vi "Start Measurement.vi"(8 "error in (no error)":errorcluster, 11 "User Interface in":refnum<class "User Interface.lvclass">) -> (0 "error out":errorcluster, 3 "User Interface out":refnum<class "User Interface.lvclass">)   [LabVIEW 2016, in "User Interface.lvlib" / "User Interface.lvclass"]
uses:
  User Interface.lvclass
  <vilib>/ActorFramework/Actor/Actor.lvclass
  Controllers/Acquisition Controller/Acquisition Controller.lvclass
  Z:/VM Shared Folder/Trace Grabber/Controllers/Abstract Controller/Abstract Controller.lvclass
  C:/Program Files (x86)/National Instruments/LabVIEW 2016/vi.lib/ActorFramework/Actor/Actor.lvclass
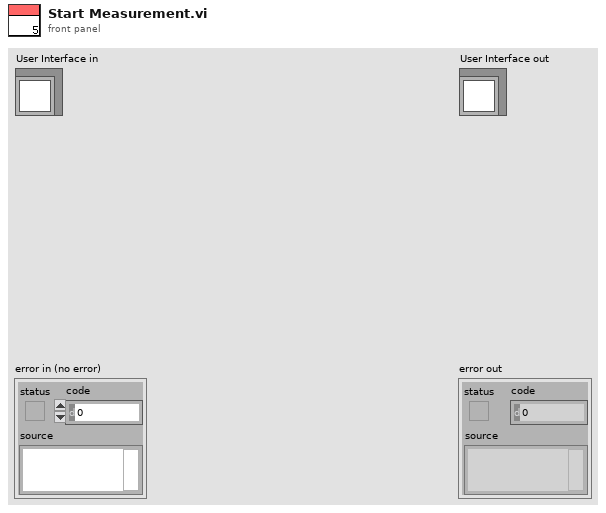
[diagram p1: front panel]
types:
  T1 = typedef "Configurations.lvlib/Configurations.lvclass/Session Handle.ctl" = refnum<data-value>
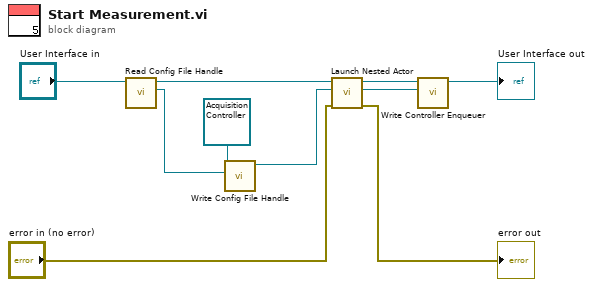
[diagram p0: block diagram]
diagram:
  n1 = call-dynamic "Read Config File Handle.vi"("User Interface in"="User Interface in") -> ("Session Handle"=w3:T1, "User Interface out"=w2:refnum<class "User Interface.lvclass">)  [unwired: 9 in]
  n2 = call-dynamic "Write Config File Handle.vi"("Session Handle"=w3, "Abstract Controller in"=refnum<class "Acquisition Controller.lvclass"> refnum ("Controllers.lvlib:Acquisition Controller.lvclass")) -> ("Abstract Controller out"=w1:refnum<class "Acquisition Controller.lvclass">)  [unwired: 9 in]
  n3 = call <vilib>:"Launch Nested Actor.vi"("error in (no error)"="error in (no error)", "Nested Actor"=w1, "Caller Actor in"=w2) -> ("error out"=→"error out":errorcluster, "Nested Actor's Enqueuer"=w10:refnum<class "Message Enqueuer.lvclass">, "Caller Actor out"=w8:refnum<class "User Interface.lvclass">)  [unwired: 6 in]
  n4 = call-dynamic "Write Controller Enqueuer.vi"("Actor Framework:Message Enqueuer"=w10, "User Interface in"=w8) -> ("User Interface out"=→"User Interface out":refnum<class "User Interface.lvclass">)  [unwired: 9 in]
